vi "ToString.vi"(0 "reference in":refnum<class "G#RemoteProxy.lvclass">, 5 "error in (no error)":errorcluster) -> (14 "reference out":refnum<class "G#RemoteProxy.lvclass">, 15 "string":string, 19 "error out":errorcluster)   [LabVIEW 2017, in "G#RemoteProxy.lvclass"]
doc: "Defines a method that allows a class to return one string as a representation of the object."
uses:
  G#RemoteProxy.lvclass
  G#DebugServer/utils/TCPCommand.ctl
  G#DebugServer/G#DebugServer.lvclass
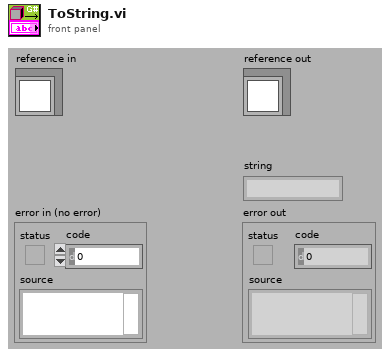
[diagram p1: front panel]
types:
  T1 = typedef "G#RemoteProxy.lvclass/ObjectAttributesProxy.ctl" = cluster{"class hierarchy":T2[], "class name":string, "lvlib hierarchy":string[], "full class name":string, "id":u32, "owner":string, "RemoteRef":refnum<class "G#Object.lvclass">, "object name":string, "attributes":variant[], "connection ID":refnum<k5>, "address":u32, "occurrence":refnum<k4>, "ProxyClassRef":refnum<class "G#RemoteProxy.lvclass">, "InMemory?":bool, "ToString":string}
  T2 = typedef "G#Object.lvclass/G#Object_ClassHierarchy.ctl" = cluster{"ClassName":string, "FullClassName":string, "ClassPath":path, "IsLeaf":bool}
  T3 = typedef "G#DebugServer.lvclass/TCPCommand.ctl" = u8
  T4 = cluster{bool, "RemoteRef":refnum<class "G#Object.lvclass">}
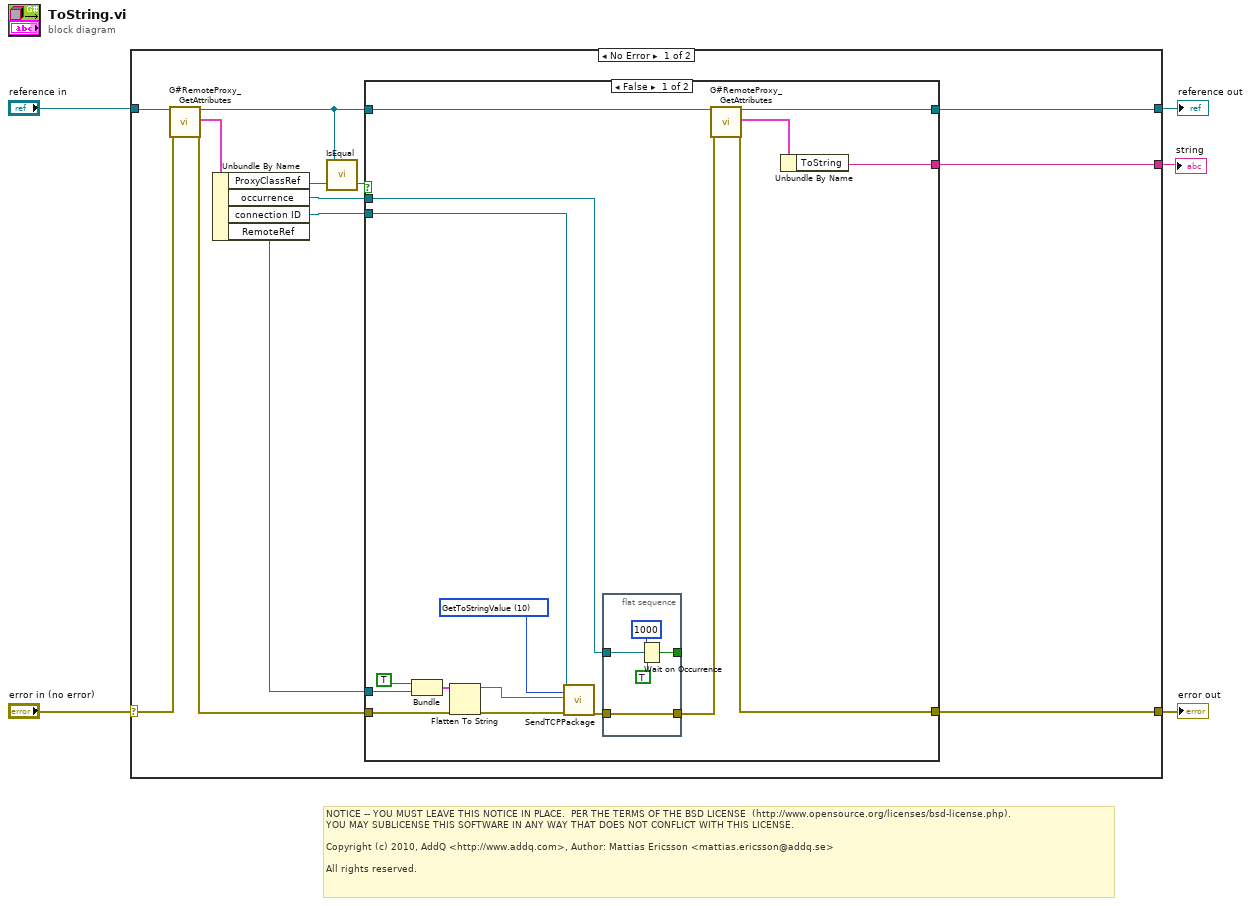
[diagram p0: block diagram]
diagram:
  # "NOTICE -- YOU MUST LEAVE THIS NOTICE IN PLACE.  PER THE TERMS OF THE BSD LICENSE  (http://www.opensource.org/licenses/bsd-license.php).\nYOU MAY SUBLICENSE THIS SOFTWARE IN ANY WAY THAT DOES NOT CONFLICT WITH THIS LICENSE.\n\nCopyright (c) 2010, AddQ <http://www.addq.com>, Author: Mattias Ericsson <mattias.ericsson@addq.se>\n\nAll rights reserved."
  n1 = case shown="No Error" "error in (no error)" {
    selector: "error in (no error)" -> [w15 w42]
    tunnel: [w10 w42] -> w4
    tunnel: [w11 w41] -> w2
    tunnel: "reference in" -> [w16 w41]
    tunnel: [w9 _] -> w1
    frame No Error {
      n2 = call "G#RemoteProxy_GetAttributes.vi"("reference in"=w16, "error in (no error)"=w15) -> ("reference out"=w7:refnum<class "G#RemoteProxy.lvclass">, "attributes"=w17:T1, "error out"=w12:errorcluster)  [unwired: 14 in, 1 out]
      n3 = Unbundle By Name(w17) -> ("occurrence"=w14:refnum<k4>, "connection ID"=w13:refnum<k5>, "RemoteRef"=w8:refnum<class "G#Object.lvclass">)  [unwired: 1 out]
      n4 = call-dynamic "IsEqual.vi"("is equal to"=w8, "reference in"=w7) -> ("is equal"=w6:bool)  [unwired: 1 out]
      n5 = case shown="False" w6 {
        tunnel: w14 -> [w32 _]
        tunnel: w13 -> [w31 _]
        tunnel: w12 -> [w29 w39]
        tunnel: [w25 w40] -> w11
        tunnel: [w23 w39] -> w10
        tunnel: [w22 _] -> w9
        tunnel: w8 -> [w19 _]
        tunnel: w7 -> [w18 w40]
        frame False {
          w30 = T3 10 items=["GarbageCollect", "GetAllObjects", "GetAllObjectsReply", "CleanUp", "G#Event", "RegisterClient", "GetAttributeValue", "GetAttributeValueReply", "GetClassAttributeValue", "GetClassAttributeValueReply", "GetToStringValue", "GetToStringValueReply", "GetClassHierarchy", "GetClassHierarchyReply", "Destroy", "RemoveClient"] ("Command")
          n6 = Bundle(TRUE, "RemoteRef"=w19) -> (w21:T4)  [unwired: 1 in]
          n7 = Flatten To String(anything=w21, error in (no error)=w29) -> (data string=w27:string, error out=w28:errorcluster)  [unwired: 2 in, 1 out]
          n8 = call "SendTCPPackage.vi"("connection ID"=w31, "command"=w30, "data"=w27, "error in (no error)"=w28) -> ("error out"=w33:errorcluster)  [unwired: 15 in]
          n9 = flat-sequence {
            tunnel: w33 -> [w36]
            tunnel: w32 -> [w38]
            tunnel: [w36] -> w24
            tunnel: [w35] -> _
            frame #0 {
              n10 = Wait on Occurrence(1:TRUE ("ignore previous (T)"), 2:w38, 3:1000 ("ms timeout (-1)")) -> (0:w35:bool)
            }
          }
          n11 = call "G#RemoteProxy_GetAttributes.vi"("reference in"=w18, "error in (no error)"=w24) -> ("reference out"=w25:refnum<class "G#RemoteProxy.lvclass">, "attributes"=w26:T1, "error out"=w23:errorcluster)  [unwired: 14 in, 1 out]
          n12 = Unbundle By Name(w26) -> ("ToString"=w22:string)
        }
        frame True {
          # "This is the class object"
        }
      }
    }
    frame Error {
    }
  }
  "error out" <- w4
  "reference out" <- w2
  "string" <- w1
